vi "Page_Shortcuts_Read.vi"(6 "ctlReferences":T1, 8 "error in (no error)":errorcluster, 11 "Class in":refnum<class "Installer.lvclass">) -> (0 "error out":errorcluster, 3 "Class out":refnum<class "Installer.lvclass">)   [LabVIEW 2020, in "Installer.lvclass"]
uses:
  <vilib>/AppBuilder/IB_Classes/Installer/Installer.lvclass
  <vilib>/AppBuilder/IB_Classes/Installer/Installer.lvclass/Installer.ctl
  <vilib>/AppBuilder/IB_Classes/Shortcut/IB_Shortcut.lvclass
  <resource>/Framework/Providers/Builds/Installer/CDK_sTypeDef_Add.ctl
  <resource>/Framework/Providers/Builds/Installer/CDK_sTypeDef_Remove.ctl
  <resource>/Framework/Providers/Builds/Installer/Pages/controls/IB_UI_Page_Shortcut_References.ctl
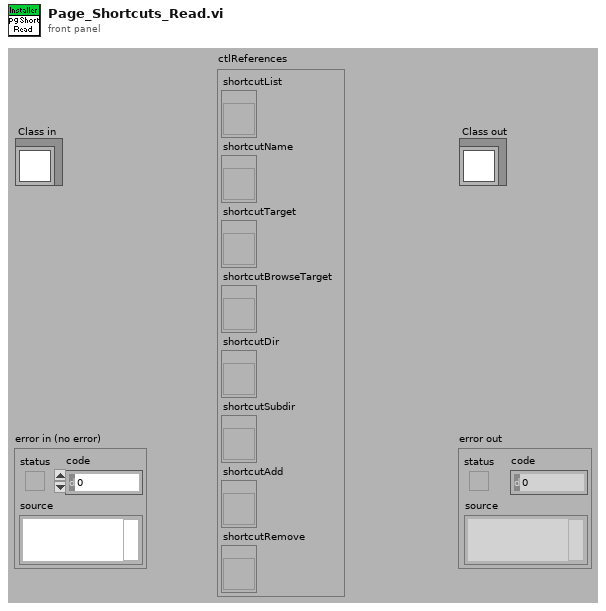
[diagram p1: front panel]
types:
  T1 = typedef "IB_UI_Page_Shortcut_References.ctl" = cluster{"shortcutList":refnum<vi>, "shortcutName":refnum<vi>, "shortcutTarget":refnum<vi>, "shortcutBrowseTarget":refnum<vi>, "shortcutDir":refnum<vi>, "shortcutSubdir":refnum<vi>, "shortcutAdd":refnum<vi>, "shortcutRemove":refnum<vi>}
  T2 = typedef "CDK_sTypeDef_ShortcutAddress.ctl" = cluster{"file":string, "shortcut":string}
  T3 = typedef "IB_Shortcut.ctl" = cluster{"name":string, "destIndex":i32, "subDir":string, "address":string}
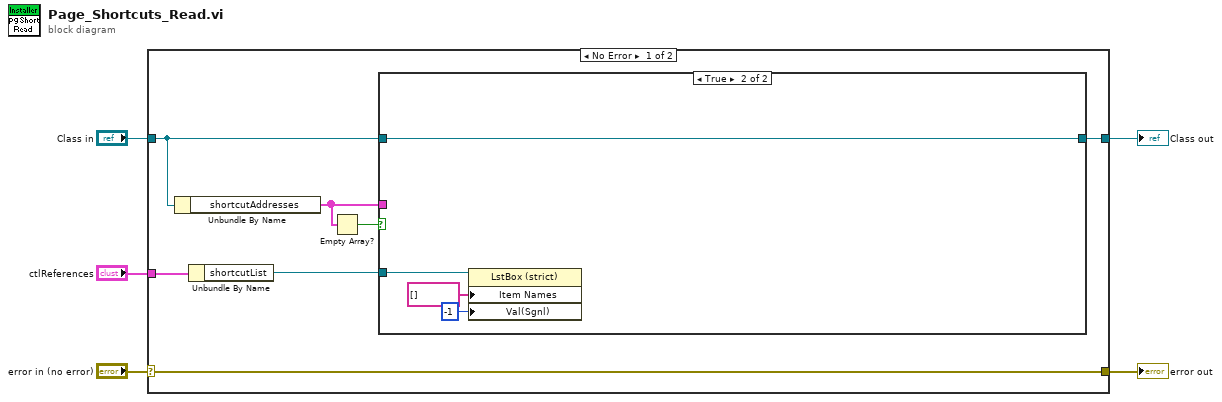
[diagram p0: block diagram]
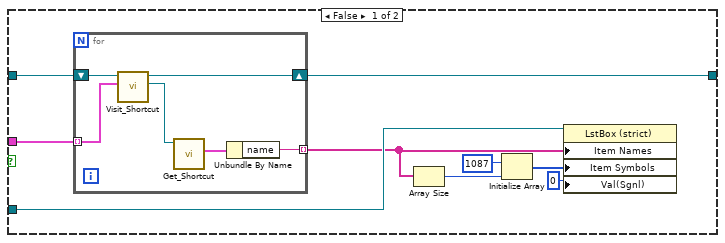
[diagram p2: hidden frame]
diagram:
  n1 = case shown="No Error" "error in (no error)" {
    selector: "error in (no error)" -> [w9 w33]
    tunnel: [w9 w33] -> w4
    tunnel: [w6 w32] -> w2
    tunnel: "Class in" -> [w7 w32]
    tunnel: "ctlReferences" -> [w12 _]
    frame No Error {
      n2 = Unbundle By Name(w7) -> ("shortcutAddresses"=w8:T2[])
      n3 = Unbundle By Name(w12) -> ("shortcutList"=w11:refnum<vi>)
      n4 = Empty Array?(array=w8) -> (empty?=w10:bool)
      n5 = case shown="True" w10 {
        tunnel: w11 -> [w18 w31]
        tunnel: w8 -> [w21 _]
        tunnel: w7 -> [w20 w29]
        tunnel: [w19 w29] -> w6
        frame False {
          n6 = for {
            tunnel: w21 -> [w22] mode=indexing
            shift-right: [w26] -> w19
            shift-left: w20 -> [w27]
            tunnel: [w23] -> w17 mode=indexing
            n7 = call <vilib>:"Visit_Shortcut.vi"("shortcut address"=w22, "Installer in"=w27) -> ("shortcut"=w25:refnum<class "IB_Shortcut.lvclass">, "Installer out"=w26:refnum<class "Installer.lvclass">)  [unwired: 2 in, 6 out]
            n8 = call <vilib>:"Get_Shortcut.vi"("Class in"=w25) -> ("data"=w24:T3)  [unwired: 1 in, 9 out]
            n9 = Unbundle By Name(w24) -> ("name"=w23:string)
          }
          n10 = Array Size(array=w17) -> (size(s)=w13:i32)
          n11 = Initialize Array(1087, w13) -> (w15:i32[])
          n12 = property class="LstBox (strict)"(reference=w18, "Item Names"=w17, "Item Symbols"=w15, "Val(Sgnl)"=0 ("Value (Signaling)")) -> ()  [unwired: 1 in, 2 out]
        }
        frame True {
          n13 = property class="LstBox (strict)"(reference=w31, "Item Names"=string[] [], "Val(Sgnl)"=-1 ("Value (Signaling)")) -> ()  [unwired: 1 in, 2 out]
        }
      }
    }
    frame Error {
    }
  }
  "error out" <- w4
  "Class out" <- w2
